vi "analyze.vi"() -> ()   [LabVIEW 2011]
uses:
  <userlib>/_OpenG.lib/dictionary/dictionary.llb/Dictionary Update (by scalar value)__ogtk.vi
  D:/gitProjects/HPTS_VNA/Data/32p_analyze.dll
  Data/32p_analyze.dll
  dataType/queueMsg.ctl
  dataType/switchMsg.ctl
  dataType/informationIn.ctl
panel:
  out "S-para Pair Name":string[](array[string])
  out "switchIndex":i32
  out "index":i32
  out "VISA COM":refnum<visa-resource-name>
  out "DAQ  Model:":T1(ring)
  out "testType":enum16{"Loss", "Next", "Fext"}(ring)
  in  "Information In":T2={"Sample PN: "="", "SampleSN:"="", "Sparam Test Item"=[], "S-para Pair Name"=[], "Length"="", "Diff Test Item Name"=["SDD21", "SDD22", "SCD21", "SCD22", "SCC11", "NEXT", "FEXT"], "Diff Test Item Name smooth"=[], "smooth point"=0.0, "limitSpec"=[], "switchIndexOffset"=0, "testType"=enum."Loss", "pairStartIndex"=0, "DAQ  Model:"=enum."NI PCI-6509", "VISA COM"="COM3", "Matrix  In"=[]}
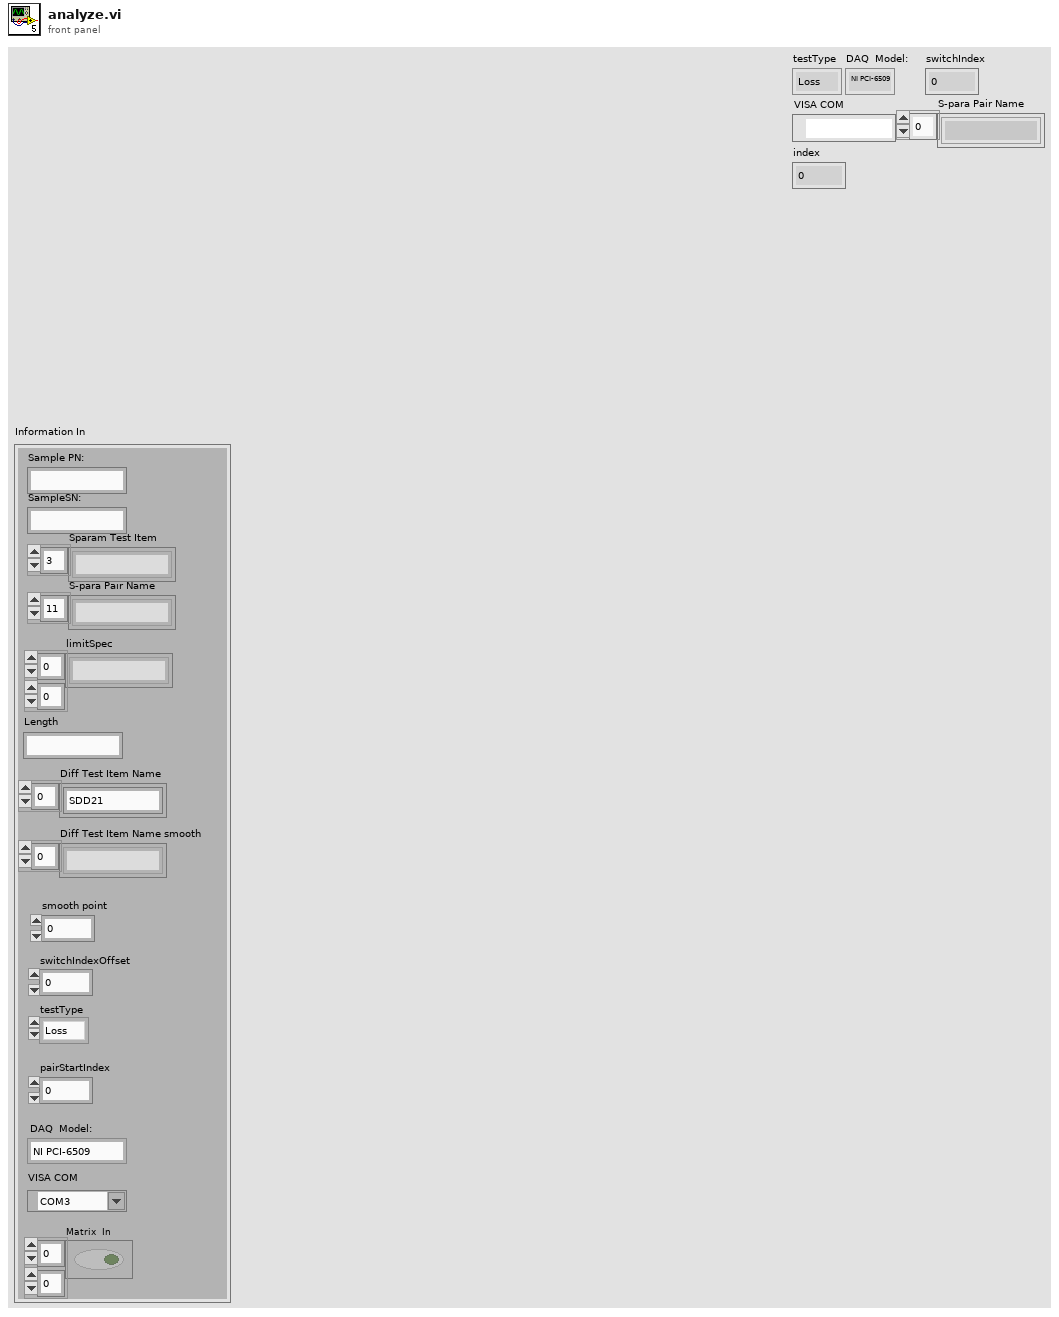
[diagram p1: front panel]
types:
  T1 = enum16{"NI PCI-6509", "LX MCU", "LX MCU_40G", "LX MCU_40G_HuaWei"}
  T2 = typedef "informationIn.ctl" = cluster{"Sample PN: ":string, "SampleSN:":string, "Sparam Test Item":string[], "S-para Pair Name":string[], "Length":string, "Diff Test Item Name":string[], "Diff Test Item Name smooth":string[], "smooth point":dbl, "limitSpec":string[][], "switchIndexOffset":i32, "testType":enum16{"Loss", "Next", "Fext"}, "pairStartIndex":i32, "DAQ  Model:":enum16{"NI PCI-6509", "LX MCU", "LX MCU_40G", "LX MCU_40G_HuaWei"}, "VISA COM":refnum<visa-resource-name>, "Matrix  In":bool[][]}
  T3 = typedef "switchMsg.ctl" = cluster{"index":i32, "pairName":string, "switchIndex":i32, "TestAction":enum16{"start", "stop", "pause", "reset"}}
  T4 = typedef "queueMsg.ctl" = cluster{"msgType":enum16{"S4P", "DATA"}, "snpPath":path, "xValue":dbl[], "yValue":dbl[][]}
  T5 = typedef "Dictionary Object RefNum__ogtk.ctl" = refnum<k1>
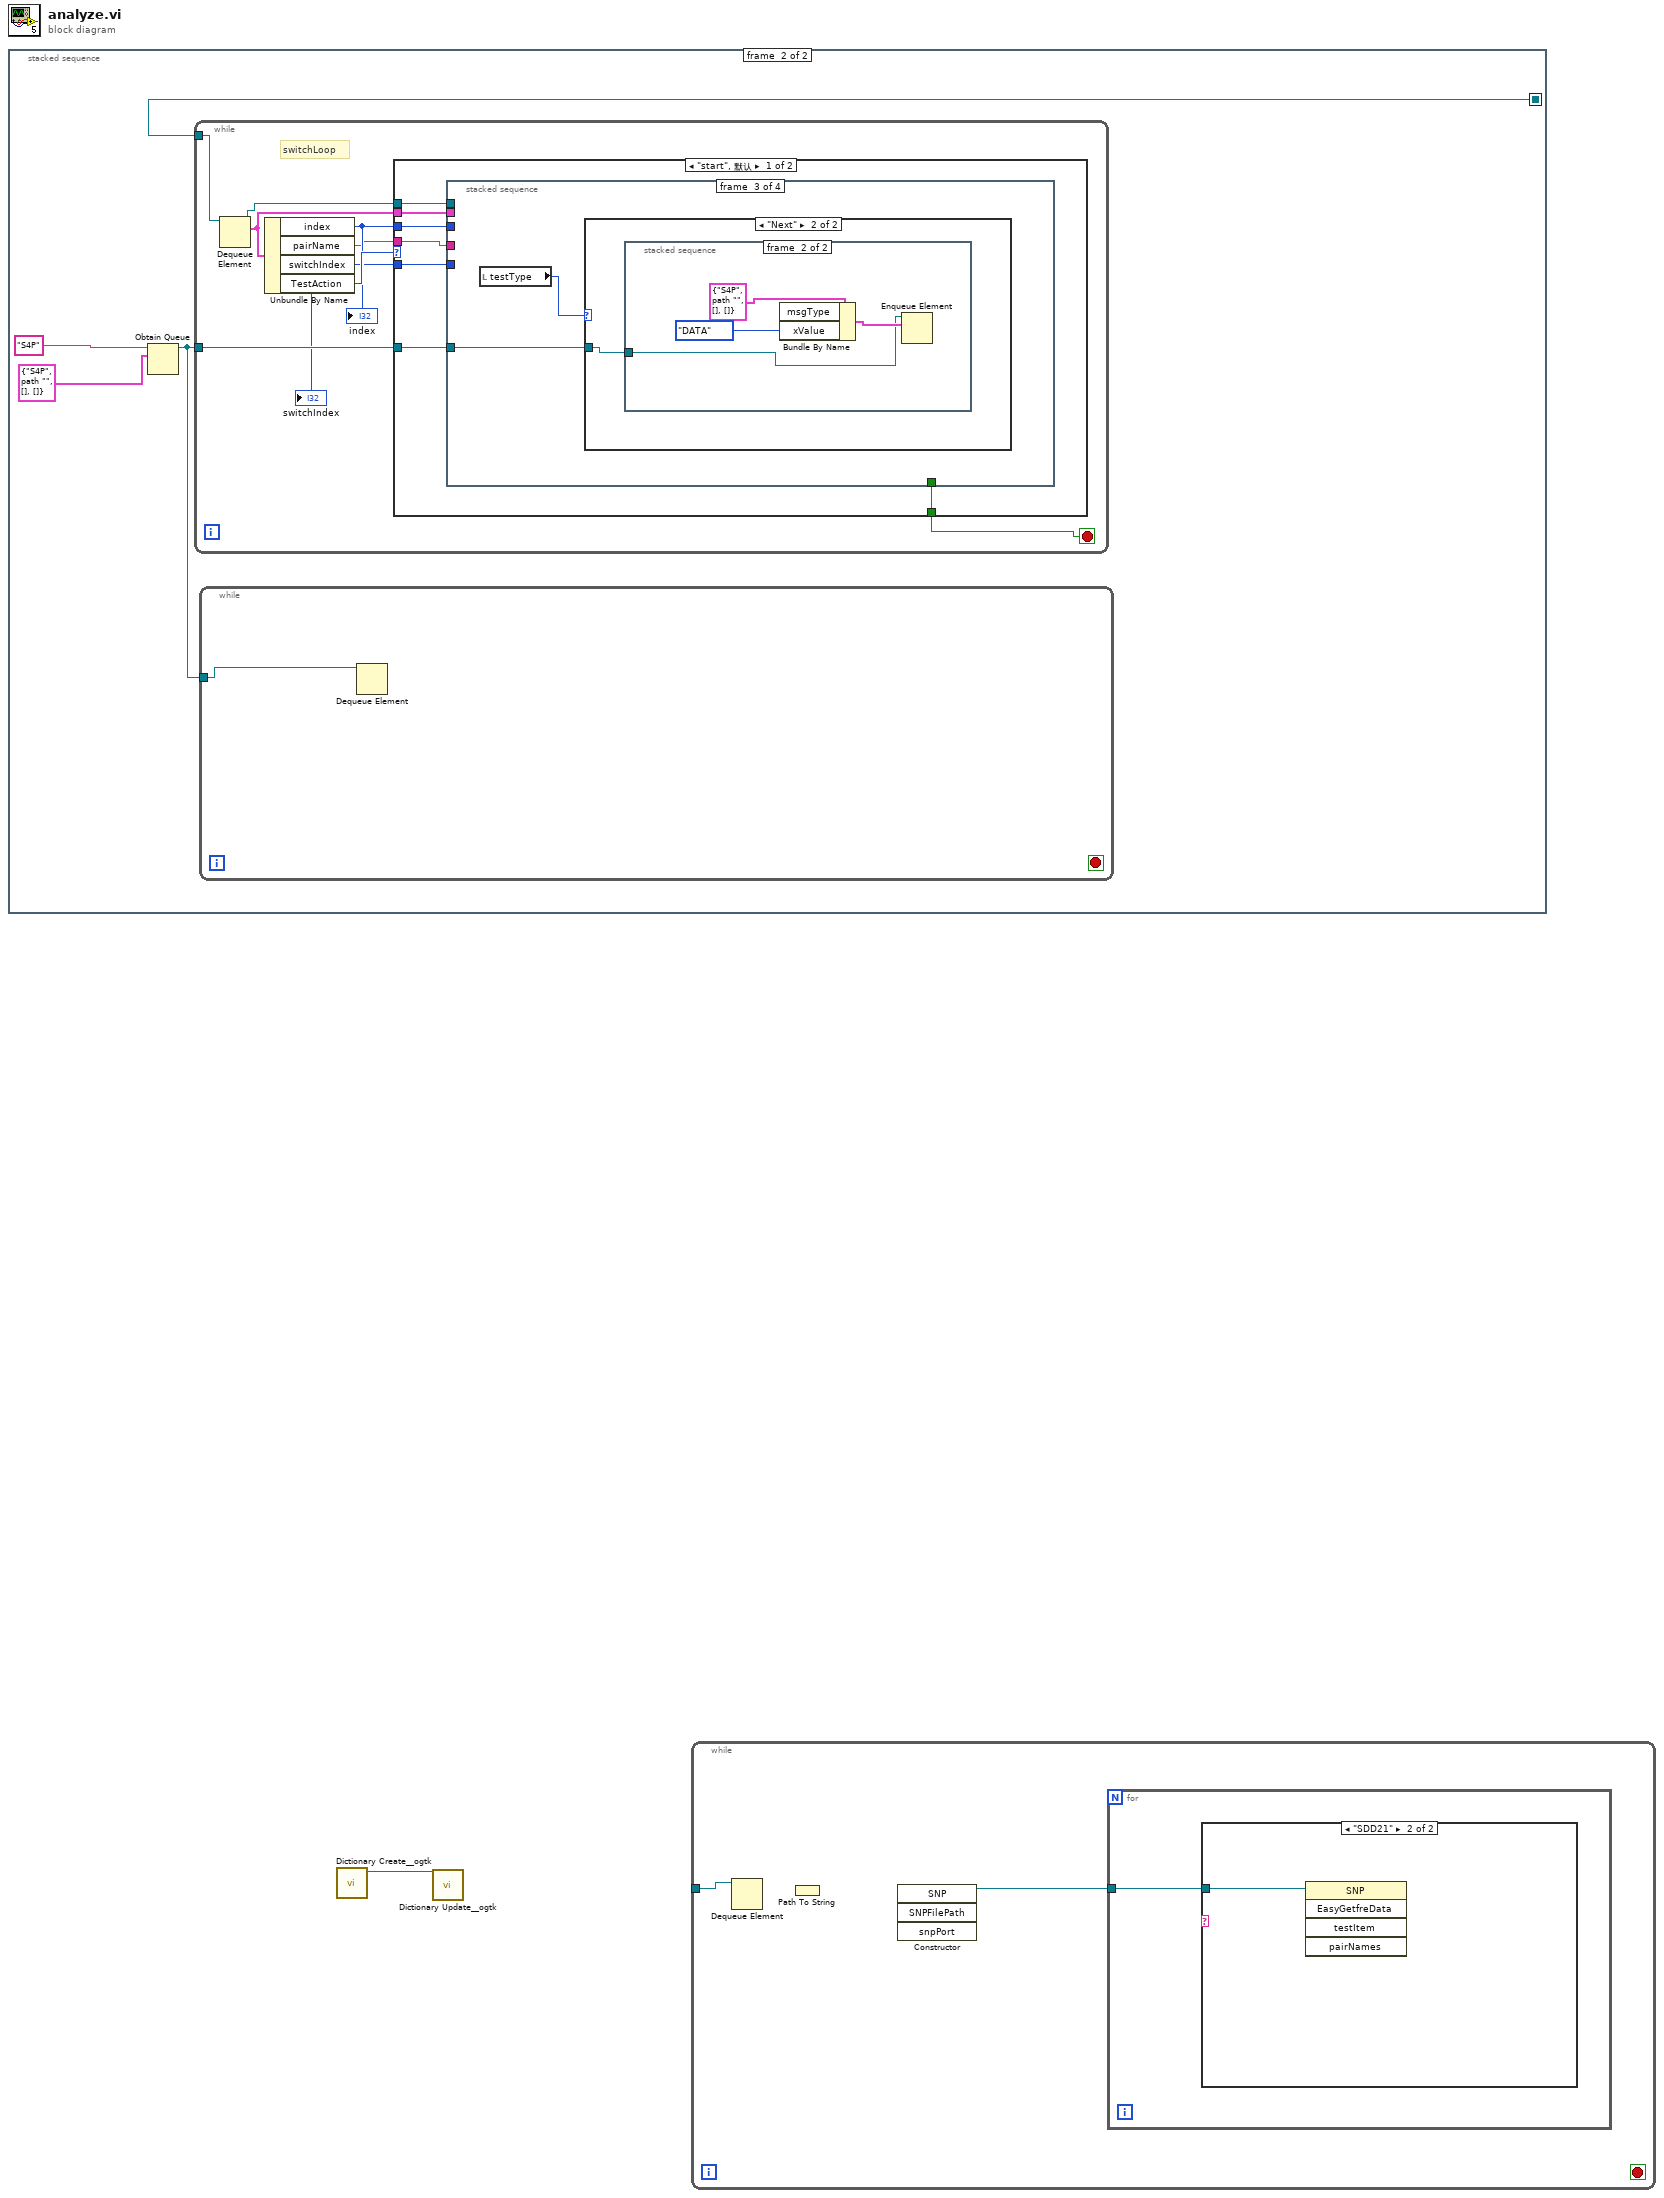
[diagram p0: block diagram]
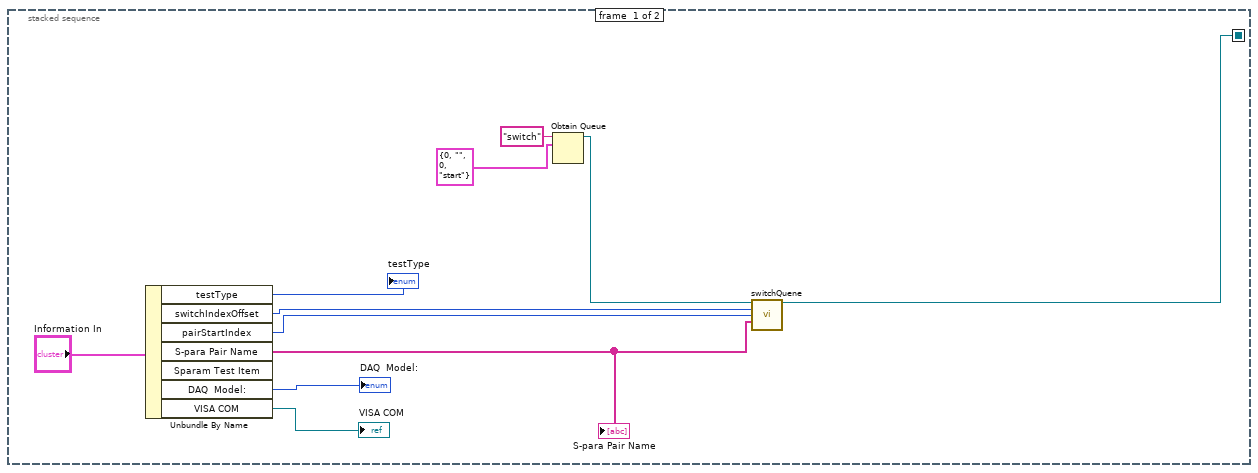
[diagram p2: hidden frame]
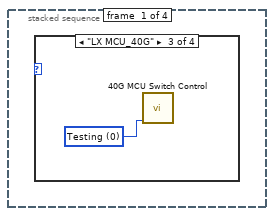
[diagram p3: hidden frame]
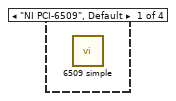
[diagram p4: hidden frame]
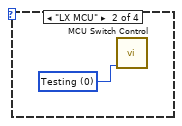
[diagram p5: hidden frame]
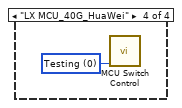
[diagram p6: hidden frame]
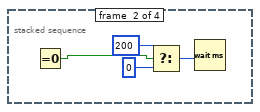
[diagram p7: hidden frame]
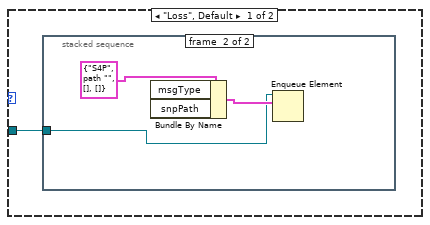
[diagram p8: hidden frame]
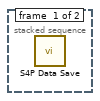
[diagram p9: hidden frame]
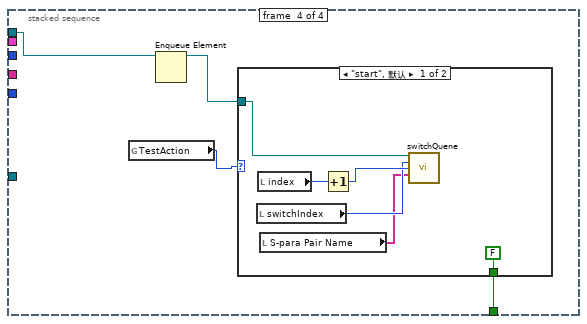
[diagram p11: hidden frame]
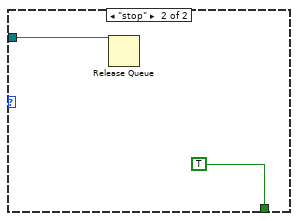
[diagram p12: hidden frame]
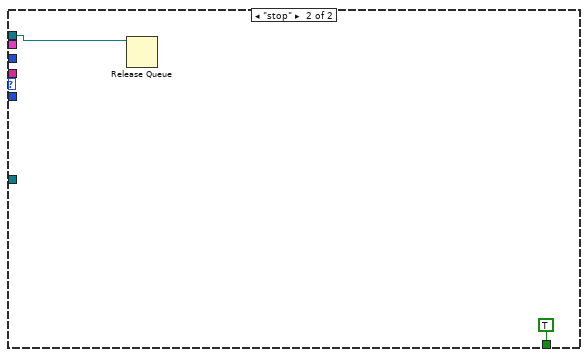
[diagram p13: hidden frame]
diagram:
  n1 = stacked-sequence {
    seq-local: [w5 _] -> [_ w16]
    frame #0 {
      n2 = Unbundle By Name("Information In") -> ("testType"=→"testType":enum16{"Loss", "Next", "Fext"}, "switchIndexOffset"=w6:i32, "pairStartIndex"=w7:i32, "S-para Pair Name"=w8:string[], "DAQ  Model:"=→"DAQ  Model:":T1, "VISA COM"=→"VISA COM":refnum<visa-resource-name>)  [unwired: 1 out]
      "S-para Pair Name" <- w8
      n3 = Obtain Queue(name (unnamed)="switch" ("名称（未命名）"), element data type=T3 {"index"=0, "pairName"="", "switchIndex"=0, "TestAction"=enum."start"} ("switchMsg")) -> (queue out=w12:refnum<queue>)  [unwired: 3 in, 2 out]
      n4 = call "switchQuene.vi"("switchQuene In"=w12, "switchIndexOffset"=w6, "pairStartIndex"=w7, "S-para Pair Name"=w8) -> ("switchQuene Out"=w5:refnum<queue>)  [unwired: 10 in, 1 out]
    }
    frame #1 {
      n5 = Obtain Queue(name (unnamed)="S4P" ("名称（未命名）"), element data type=T4 {"msgType"=enum."S4P", "snpPath"=path "", "xValue"=[], "yValue"=[]} ("queueMsg")) -> (queue out=w13:refnum<queue>)  [unwired: 3 in, 2 out]
      n6 = while {
        tunnel: w16 -> [w26]
        tunnel: w13 -> [w24]
        stop <- w18 stop-if-true
        # "switchLoop"
        n7 = Dequeue Element(queue=w26) -> (queue out=w22:refnum<queue>, element=w23:T3)  [unwired: 2 in, 2 out]
        n8 = Unbundle By Name(w23) -> ("index"=w21:i32, "pairName"=w20:string, "switchIndex"=w19:i32, "TestAction"=w25:enum16{"start", "stop", "pause", "reset"})
        "index" <- w21
        "switchIndex" <- w19
        n9 = case shown="\"start\", 默认" w25 {
          tunnel: w24 -> [w33 _]
          tunnel: w23 -> [w32 _]
          tunnel: w22 -> [w31 w64]
          tunnel: w21 -> [w30 _]
          tunnel: w20 -> [w29 _]
          tunnel: w19 -> [w28 _]
          tunnel: [w27 TRUE] -> w18
          frame "start", Default {
            n10 = stacked-sequence {
              tunnel: w33 -> [_ _ w41 _]
              tunnel: w32 -> [_ _ _ _]
              tunnel: w31 -> [_ _ _ w55]
              tunnel: w30 -> [_ _ _ _]
              tunnel: w29 -> [_ _ _ _]
              tunnel: w28 -> [_ _ _ _]
              tunnel: [_ _ _ w52] -> w27
              frame #0 {
                n11 = case shown="\"LX MCU_40G\"" {
                  selector: _ -> [_ _ _ _]
                  frame "NI PCI-6509", Default {
                    n12 = call "6509 simple.vi"() -> ()  [unwired: 7 in, 1 out]
                  }
                  frame "LX MCU" {
                    w34 = u16 0 items=["Testing", "Close All"] ("Function")
                    n13 = call "MCU Switch Control.vi"("Function"=w34) -> ()  [unwired: 10 in, 1 out]
                  }
                  frame "LX MCU_40G" {
                    w35 = u16 0 items=["Testing", "Close All"] ("Function")
                    n14 = call "40G MCU Switch Control.vi"("Function"=w35) -> ()  [unwired: 10 in, 1 out]
                  }
                  frame "LX MCU_40G_HuaWei" {
                    w36 = u16 0 items=["Testing", "Close All"] ("Function")
                    n15 = call "MCU Switch Control.vi"("Function"=w36) -> ()  [unwired: 10 in, 1 out]
                  }
                }
              }
              frame #1 {
                n16 = Equal To 0?() -> (x = 0?=w40:bool)  [unwired: 1 in]
                n17 = Select(t=200, s=w40, f=0) -> (s? t:f=w37:i32)
                n18 = Wait (ms)(milliseconds to wait=w37) -> ()  [unwired: 1 out]
              }
              frame #2 {
                n19 = local read "testType"() -> (w42:enum16{"Loss", "Next", "Fext"})
                n20 = case shown="\"Next\"" w42 {
                  tunnel: w41 -> [w43 w47]
                  frame "Loss", Default {
                    n21 = stacked-sequence {
                      tunnel: w43 -> [_ w44]
                      frame #0 {
                        n22 = call "S4P Data Save.vi"() -> ()  [unwired: 17 in, 3 out]
                      }
                      frame #1 {
                        n23 = Bundle By Name(cluster=T4 {"msgType"=enum."S4P", "snpPath"=path "", "xValue"=[], "yValue"=[]} ("queueMsg")) -> (w45:T4)  [unwired: 2 in]
                        n24 = Enqueue Element(queue=w44, element=w45) -> ()  [unwired: 2 in, 3 out]
                      }
                    }
                  }
                  frame "Next" {
                    n25 = stacked-sequence {
                      tunnel: w47 -> [_ w49]
                      frame #0 {
                      }
                      frame #1 {
                        n26 = Bundle By Name(cluster=T4 {"msgType"=enum."S4P", "snpPath"=path "", "xValue"=[], "yValue"=[]} ("queueMsg"), "msgType"=enum16{"S4P", "DATA"}."DATA") -> (w50:T4)  [unwired: 1 in]
                        n27 = Enqueue Element(queue=w49, element=w50) -> ()  [unwired: 2 in, 3 out]
                      }
                    }
                  }
                }
              }
              frame #3 {
                n28 = global read "全局.vi" "TestAction"() -> (w54:enum16{"start", "stop", "pause", "reset"})
                n29 = Enqueue Element(queue=w55) -> (queue out=w53:refnum<queue>)  [unwired: 3 in, 2 out]
                n30 = case shown="\"start\", 默认" w54 {
                  tunnel: w53 -> [w61 w63]
                  tunnel: [FALSE TRUE] -> w52
                  frame "start", Default {
                    n31 = local read "switchIndex"() -> (w58:i32)
                    n32 = local read "index"() -> (w59:i32)
                    n33 = local read "S-para Pair Name"() -> (w57:string[])
                    n34 = Increment(x=w59) -> (x+1=w60:i32)
                    n35 = call "switchQuene.vi"("switchQuene In"=w61, "switchIndexOffset"=w58, "pairStartIndex"=w60, "S-para Pair Name"=w57) -> ()  [unwired: 10 in, 2 out]
                  }
                  frame "stop" {
                    n36 = Release Queue(queue=w63) -> ()  [unwired: 2 in, 3 out]
                  }
                }
              }
            }
          }
          frame "stop" {
            n37 = Release Queue(queue=w64) -> ()  [unwired: 2 in, 3 out]
          }
        }
      }
      n38 = while {
        tunnel: w13 -> [w17]
        stop <- _ stop-if-true
        n39 = Dequeue Element(queue=w17) -> ()  [unwired: 2 in, 4 out]
      }
    }
  }
  n40 = call <userlib>:"Dictionary Create__ogtk.vi"() -> ("dictionary out"=w1:T5)  [unwired: 10 in, 1 out]
  n41 = call-poly <userlib>:"Dictionary Update__ogtk.vi"("dictionary"=w1) -> ()  [unwired: 8 in, 3 out]
  n42 = while {
    tunnel: _ -> [w67]
    stop <- _ stop-if-true
    n43 = Dequeue Element(queue=w67) -> ()  [unwired: 2 in, 4 out]
    n44 = Path To String() -> ()  [unwired: 1 in, 1 out]
    n45 = constructor class="SNP"() -> (reference out=w66:refnum<k24>)  [unwired: 5 in, 4 out]
    n46 = for {
      tunnel: w66 -> [w68]
      n47 = case shown="\"SDD21\"" {
        selector: _ -> [_ _]
        tunnel: w68 -> [_ w69]
        frame "假", Default {
        }
        frame "SDD21" {
          n48 = invoke class="SNP" method="EasyGetfreData"(reference=w69) -> ()  [unwired: 4 in, 5 out]
        }
      }
    }
  }
